vi "Increase Count.vi"(8 "error in (no error)":errorcluster, 10 "Amount":dbl=1.0, 11 "Worker in":refnum<class "Worker.lvclass">) -> (0 "error out":errorcluster, 3 "Worker out":refnum<class "Worker.lvclass">)   [LabVIEW 2023, in "Worker.lvlib" / "Worker.lvclass"]
doc: "Increases the worker's count of tasks completed by <b>Amount</b>."
uses:
  Worker.lvclass
  Worker.lvclass/Worker.ctl
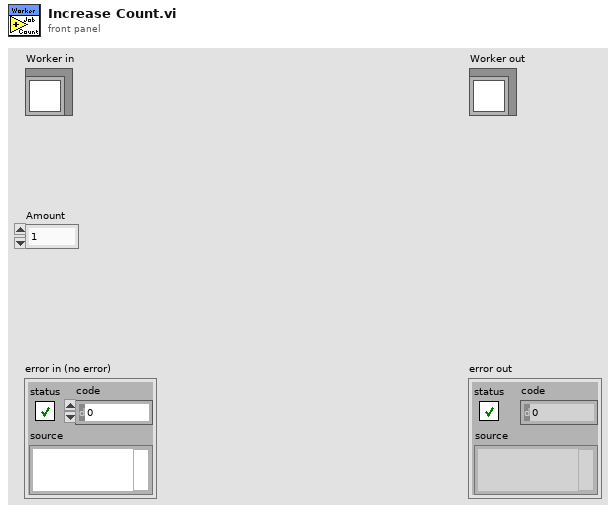
[diagram p1: front panel]
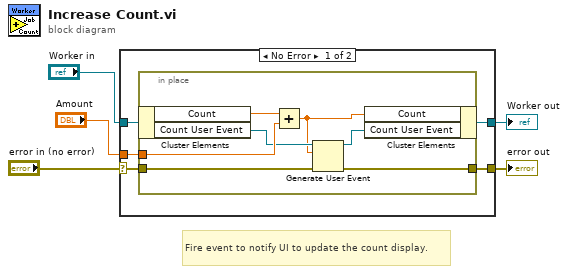
[diagram p0: block diagram]
diagram:
  # "Fire event to notify UI to update the count display."
  n1 = case shown="No Error" "error in (no error)" {
    selector: "error in (no error)" -> [w7 w19]
    tunnel: [w6 w19] -> w4
    tunnel: [w10 w18] -> w2
    tunnel: "Worker in" -> [w8 w18]
    tunnel: "Amount" -> [w9 _]
    frame No Error {
      n2 = in-place "In Place Element Structure" {
        in-place-border: w9 -> [w16]
        in-place-border: w7 -> [w12]
        in-place-border: [w11] -> w6
        n3 = in-place-cluster #1 ("Unbundle / Bundle Elements")(w8) -> ("Count"=w17:dbl, "Count User Event"=w15:refnum<user-event>)
        n4 = Add(x=w17, y=w16) -> (x+y=w13:dbl)
        n5 = Generate User Event(user event=w15, event data cluster=w13, error in=w12) -> (user event out=w14:refnum<user-event>, error out=w11:errorcluster)  [unwired: 1 in]
        n6 = in-place-cluster #1 ("Unbundle / Bundle Elements")("Count"=w13, "Count User Event"=w14) -> (w10:refnum<class "Worker.lvclass">)
      }
    }
    frame Error {
    }
  }
  "error out" <- w4
  "Worker out" <- w2
